vi "Run 1.vi"   [LabVIEW 2016]
types:
  T1 = typedef "LVHSConnector.ctl" = refnum<class "BrickReference.lvclass">
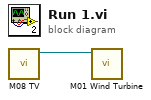
[diagram p0: block diagram]
diagram:
  n1 = call "M08 TV.vi"() -> ("EV3 out"=w1:T1)  [unwired: 11 in]
  n2 = call "M01 Wind Turbine.vi"("EV3 in"=w1) -> ()  [unwired: 11 in]
